vi "ABR3-Analyze With User Window.vi"(0 "Analysis":T1, 7 "Tmax (ms)":dbl, 11 "error in":errorcluster) -> (4 "Analysis Out":T1, 15 "error out":errorcluster)   [LabVIEW 2020]
uses:
  TypeDefs/ABR3-Analysis State.ctl
  Threshold Estimation VIs/ABR3-Threshold Estimation Result.ctl
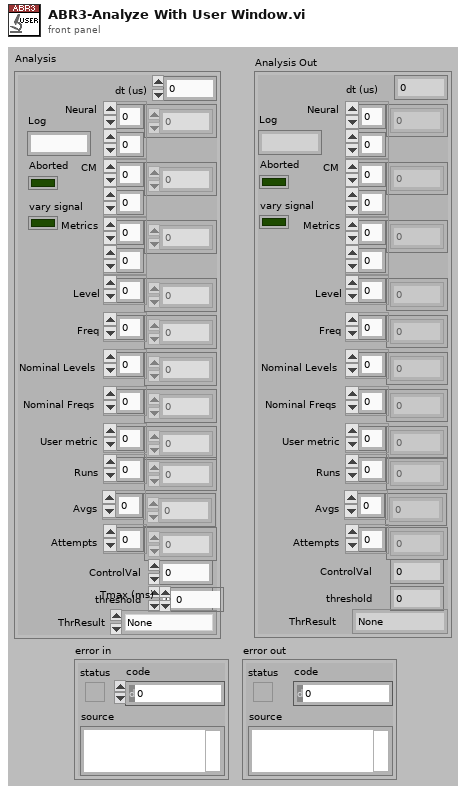
[diagram p1: front panel]
types:
  T1 = typedef "ABR3-Analysis State.ctl" = cluster{"dt (us)":dbl, "Neural":dbl[][], "CM":dbl[][], "Metrics":dbl[][], "Level":dbl[], "Freq":dbl[], "Nominal Levels":dbl[], "Nominal Freqs":dbl[], "User metric":dbl[], "Runs":i32[], "Avgs":i32[], "Attempts":i32[], "Log":string, "Aborted":bool, "ControlVal":dbl, "threshold":dbl, "vary signal":bool, "ThrResult":T2}
  T2 = typedef "ABR3-Threshold Estimation Result.ctl" = enum16{"None", "Power", "Sigmoid", "Power (noisy)", "Suprathreshold", "Invalid"}
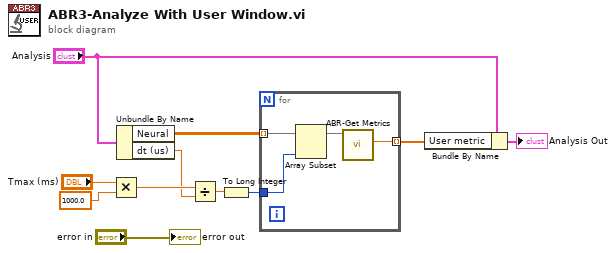
[diagram p0: block diagram]
diagram:
  n1 = Multiply(x="Tmax (ms)", y=1000.0) -> (x*y=w7:dbl)
  n2 = Unbundle By Name("Analysis") -> ("Neural"=w11:dbl[][], "dt (us)"=w6:dbl)
  n3 = Divide(x=w7, y=w6) -> (x/y=w5:dbl)
  n4 = To Long Integer(number=w5) -> (32bit integer=w4:i32)
  n5 = for {
    tunnel: w11 -> [w15] mode=indexing
    tunnel: w4 -> [w13]
    tunnel: [w12] -> w2 mode=indexing
    n6 = Array Subset(array=w15, length=w13) -> (w14:dbl[])  [unwired: 1 in]
    n7 = call "ABR-Get Metrics.vi"("Data in"=w14) -> ("spread value"=w12:dbl)  [unwired: 8 in, 2 out]
  }
  n8 = Bundle By Name(cluster="Analysis", "User metric"=w2) -> (→"Analysis Out":T1)
  "error out" <- "error in"
